vi "SwerveLatchGoalAngle.vi"(1 "Raw Goal Angle":dbl format="%#_13g", 2 "In Deadband":bool) -> (0 "Latched Goal Angle":dbl)   [LabVIEW 2020]
doc: "Latches the goal azimuth angle when the driver releases the stick. This prevents the modules from slewing to a new orientation and jerking the robot."
uses:
  Auto/Auto Commands/4265 Drive Path/sensors.vi
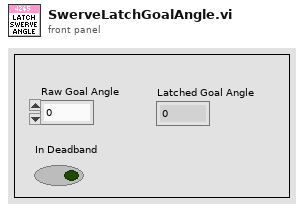
[diagram p1: front panel]
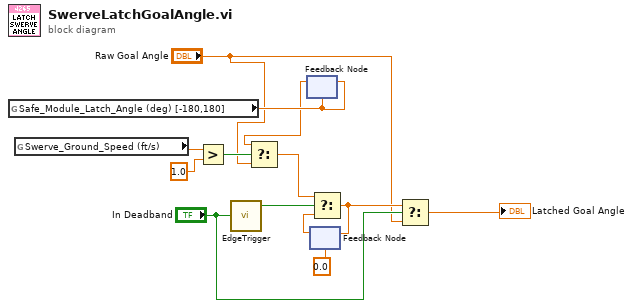
[diagram p0: block diagram]
diagram:
  n1 = global read "sensors.vi" "Safe_Module_Latch_Angle (deg) [-180,180]"() -> (w7:dbl)
  n2 = global read "sensors.vi" "Swerve_Ground_Speed (ft/s)"() -> (w6:dbl)
  n3 = Greater?(x=w6, y=1.0) -> (0:w5:bool)
  n4 = call "EdgeTrigger.vi"("Input Signal"="In Deadband") -> ("Rising Edge Trigger"=w13:bool)  [unwired: 2 out]
  n5 = feedback-in #1(w7) -> ()
  n6 = feedback #1(w7) -> (w3:dbl)
  n7 = Select(t=w3, s=w5, f="Raw Goal Angle") -> (s? t:f=w1:dbl)
  n8 = feedback #2(0.0) -> (w11:dbl)
  n9 = Select(t=w1, s=w13, f=w11) -> (s? t:f=w10:dbl)
  n10 = feedback-in #2(w10) -> ()
  n11 = Select(t=w10, s="In Deadband", f="Raw Goal Angle") -> (s? t:f=→"Latched Goal Angle":dbl)
